vi "Interpolation_KNRm.vi"(8 "error in (no error)":errorcluster, 10 "Move":T1, 11 "KNR in":T2) -> (0 "error out":errorcluster, 2 "Alpha":dbl, 3 "KNR out":T2)   [LabVIEW 2013]
uses:
  <userlib>/KNR OS 3.0 LabVIEW Toolkit/Type Definition/KNR3 Reference.ctl
  <userlib>/_FPGA Interface Advanced Tools/FPGA Interface Base/FPGA Interface Base.lvclass
  <userlib>/KNR OS 3.0 LabVIEW Toolkit/Type Definition/Resource.ctl
  Global_KNRm.vi
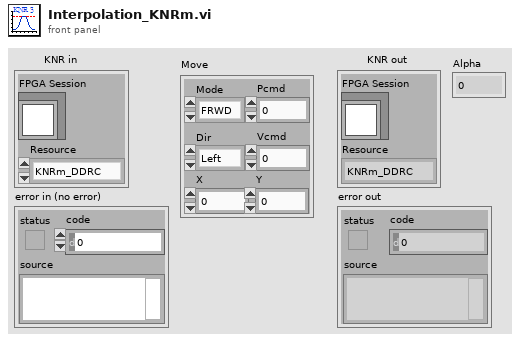
[diagram p1: front panel]
types:
  T1 = cluster{"Mode":enum16{"FRWD", "TURFIX", "TURNOF", "CIRCULAR"}, "Dir":enum16{"Left", "Right"}, "Pcmd":dbl, "Vcmd":dbl, "X":dbl, "Y":dbl}
  T2 = typedef "KNR3 Reference.ctl" = cluster{"FPGA Session":refnum<class "FPGA Interface Base.lvclass">, "Resource":T3}
  T3 = typedef "Resource.ctl" = enum16{"KNRm_DDRC", "KNRm_DDDD", "KNRm_DDDR", "KNRm_DDDC", "KNR"}
  T4 = cluster{"Nacc":i32, "deg":dbl, "cnt":i32, "Tacc":dbl, "Lest":dbl, "Ocmd":dbl, "Nc":i32, "Lmin":dbl, "Tcmd":dbl, "Tc":dbl, "Type":i32, "itrflg":i32}
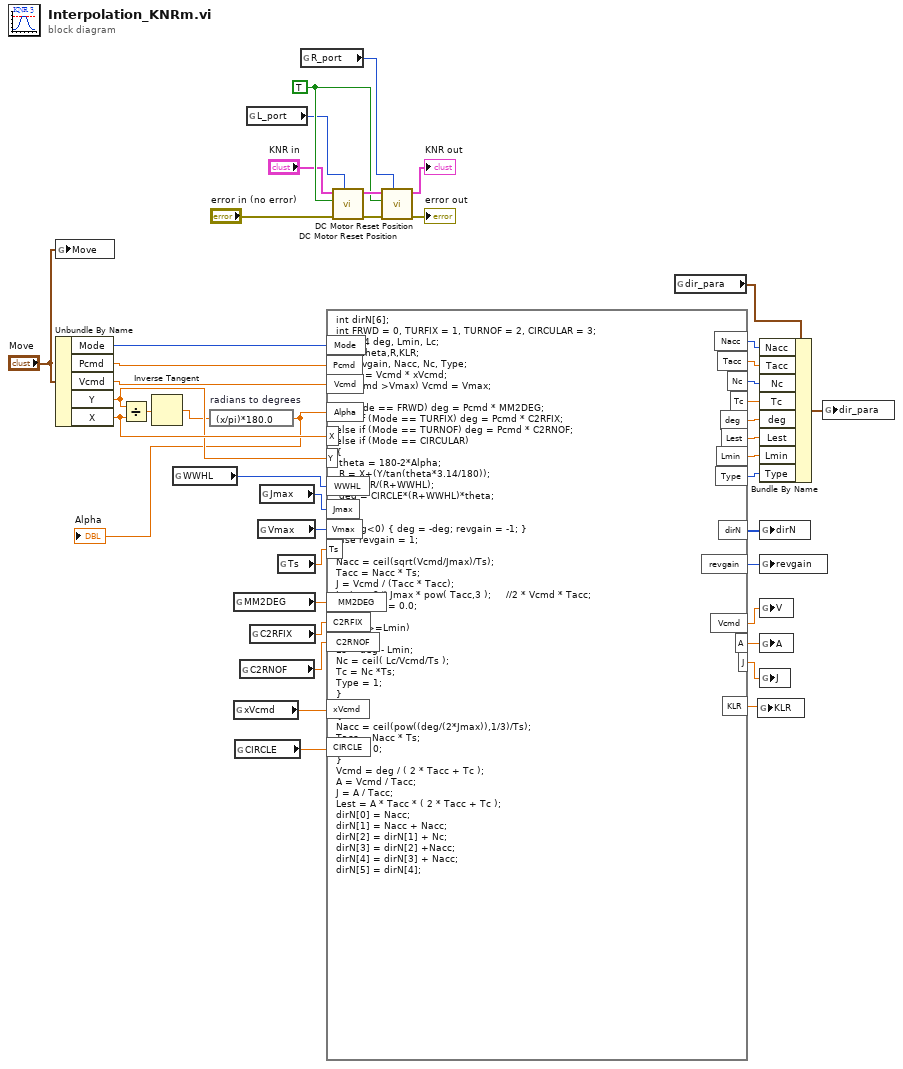
[diagram p0: block diagram]
diagram:
  w41 = TRUE ("Reset(F)")
  n1 = global write "Global_KNRm.vi" "Move"("Move") -> ()
  n2 = Unbundle By Name("Move") -> ("Mode"=w33:enum16{"FRWD", "TURFIX", "TURNOF", "CIRCULAR"}, "Pcmd"=w32:dbl, "Vcmd"=w31:dbl, "Y"=w6:dbl, "X"=w7:dbl)
  n3 = Divide(x=w6, y=w7) -> (x/y=w8:dbl)
  n4 = Inverse Tangent(1:w8) -> (0:w3:dbl)
  n5 = global read "Global_KNRm.vi" "WWHL"() -> (w5:i32)
  n6 = expression code="(x/pi)*180.0" "radians to degrees"(w3) -> (w2:dbl)
  "Alpha" <- w2
  n7 = global read "Global_KNRm.vi" "MM2DEG"() -> (w27:dbl)
  n8 = global read "Global_KNRm.vi" "xVcmd"() -> (w9:dbl)
  n9 = global read "Global_KNRm.vi" "CIRCLE"() -> (w4:dbl)
  n10 = global read "Global_KNRm.vi" "C2RNOF"() -> (w25:dbl)
  n11 = global read "Global_KNRm.vi" "L_port"() -> (w40:i8)
  n12 = global read "Global_KNRm.vi" "C2RFIX"() -> (w26:dbl)
  n13 = global read "Global_KNRm.vi" "Vmax"() -> (w29:i32)
  n14 = global read "Global_KNRm.vi" "Jmax"() -> (w30:i32)
  n15 = global read "Global_KNRm.vi" "Ts"() -> (w28:dbl)
  n16 = global read "Global_KNRm.vi" "R_port"() -> (w39:i8)
  n17 = formula code="int dirN[6];\nint FRWD = 0, TURFIX = 1, TURNOF = 2, CIRCULAR = 3;\nfloat64 deg, Lmin, Lc;\nfloat theta,R,KLR;\nint revgain, Nacc, Nc, Type;\nVcmd = Vcmd * xVcmd;\nif ( Vcmd >Vmax) Vcmd = Vmax;\n\nif (Mode == FRWD) deg = Pcmd * MM2DEG;\nelse if (Mode == TURFIX) deg = Pcmd * C2RFIX;\nelse if (Mode == TURNOF) deg = Pcmd * C2RNOF;\nelse if (Mode == CIRCULAR)\n{\n theta = 180-2*Alpha;\n R = X+(Y/tan(theta*3.14/180));\n KLR = R/(R+WWHL);\n deg = CIRCLE*(R+WWHL)*theta;\n}\n\nif (deg<0) { deg = -deg; revgain = -1; }\nelse revgain = 1;\n\nNacc = ceil(sqrt(Vcmd/Jmax)/Ts);\nTacc = Nacc * Ts;\nJ = Vcmd / (Tacc * Tacc);\nLmin = 2 * Jmax * pow( Tacc,3 );     //2 * Vcmd * Tacc;\nNc = 0; Tc = 0.0;\n\nif (deg>=Lmin)\n{\nLc = deg - Lmin;\nNc = ceil( Lc/Vcmd/Ts );\nTc = Nc *Ts;\nType = 1;\n}\nelse\n{\nNacc = ceil(pow((deg/(2*Jmax)),1/3)/Ts);\nTacc = Nacc * Ts;\nType = 0;\n}\nVcmd = deg / ( 2 * Tacc + Tc );\nA = Vcmd / Tacc;\nJ = A / Tacc;\nLest = A * Tacc * ( 2 * Tacc + Tc );\ndirN[0] = Nacc;\ndirN[1] = Nacc + Nacc;\ndirN[2] = dirN[1] + Nc;\ndirN[3] = dirN[2] +Nacc;\ndirN[4] = dirN[3] + Nacc;\ndirN[5] = dirN[4];"("Mode"=w33, "Pcmd"=w32, "Vcmd"=w31, "Jmax"=w30, "Vmax"=w29, "Ts"=w28, "MM2DEG"=w27, "C2RFIX"=w26, "C2RNOF"=w25, "xVcmd"=w9, "Alpha"=w2, "X"=w7, "Y"=w6, "WWHL"=w5, "CIRCLE"=w4) -> ("Nacc"=w22:i32, "Tacc"=w21:dbl, "Nc"=w20:i32, "Tc"=w19:dbl, "deg"=w18:dbl, "Lest"=w17:dbl, "Lmin"=w16:dbl, "Type"=w15:i32, "dirN"=w14:i32[], "revgain"=w13:i32, "Vcmd"=w12:dbl, "A"=w11:dbl, "J"=w10:dbl, "KLR"=w1:dbl)
  n18 = call <userlib>:"DC Motor Reset Position.vi"("Port (DS1)"=w40, "error in (no error)"="error in (no error)", "Reset(F)"=w41, "KNR in"="KNR in") -> ("error out"=w42:errorcluster, "KNR out"=w43:T2)  [unwired: 6 in]
  n19 = call <userlib>:"DC Motor Reset Position.vi"("Port (DS1)"=w39, "error in (no error)"=w42, "Reset(F)"=w41, "KNR in"=w43) -> ("error out"=→"error out":errorcluster, "KNR out"=→"KNR out":T2)  [unwired: 6 in]
  n20 = global read "Global_KNRm.vi" "dir_para"() -> (w24:T4)
  n21 = global write "Global_KNRm.vi" "KLR"(w1) -> ()
  n22 = Bundle By Name(cluster=w24, "Nacc"=w22, "Tacc"=w21, "Nc"=w20, "Tc"=w19, "deg"=w18, "Lest"=w17, "Lmin"=w16, "Type"=w15) -> (w23:T4)
  n23 = global write "Global_KNRm.vi" "dirN"(w14) -> ()
  n24 = global write "Global_KNRm.vi" "revgain"(w13) -> ()
  n25 = global write "Global_KNRm.vi" "V"(w12) -> ()
  n26 = global write "Global_KNRm.vi" "A"(w11) -> ()
  n27 = global write "Global_KNRm.vi" "J"(w10) -> ()
  n28 = global write "Global_KNRm.vi" "dir_para"(w23) -> ()
